vi "DebugMessage.vi"(11 "CommandVI":string) -> (3 "StartDebug":bool)   [LabVIEW 2021, in "YActor.lvclass"]
uses:
  YActor.lvclass
  Debug Messages.vi
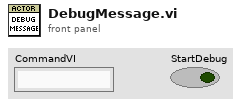
[diagram p1: front panel]
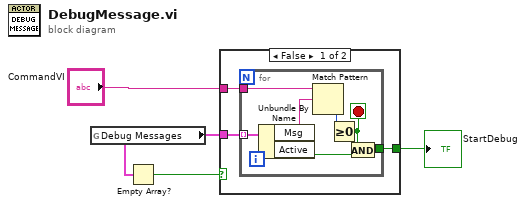
[diagram p0: block diagram]
diagram:
  n1 = global read "Debug Messages.vi" "Debug Messages"() -> (w3:cluster{"Msg":string, "Active":bool}[])
  n2 = Empty Array?(array=w3) -> (empty?=w1:bool)
  n3 = case shown="False" w1 {
    tunnel: w3 -> [w7 _]
    tunnel: "CommandVI" -> [w6 _]
    tunnel: [w5 _] -> w2
    frame False {
      n4 = for {
        tunnel: w7 -> [w14] mode=indexing
        tunnel: w6 -> [w12]
        tunnel: [w8] -> w5
        stop <- w9 stop-if-true
        n5 = Unbundle By Name(w14) -> ("Msg"=w13:string, "Active"=w10:bool)
        n6 = Match Pattern(string=w12, regular expression=w13) -> (offset past match=w11:i32)  [unwired: 1 in, 3 out]
        n7 = Greater Or Equal To 0?(x=w11) -> (x >= 0?=w9:bool)
        n8 = And(x=w9, y=w10) -> (x .and. y?=w8:bool)
      }
    }
    frame True {
    }
  }
  "StartDebug" <- w2
